vi "AppendToParentsList.vi"(10 "Dependendent TypeDefs wParents (in)":T1[](array[typedef]), 11 "Dependendent TypeDef wParents":T1) -> (2 "Dependendent TypeDefs wParents (out)":T1[](array[typedef]))   [LabVIEW 2013, in "DiscoverCommonTypeDefCallers.lvlib"]
uses:
  DiscoverCommonTypeDefCallers.lvlib
  DependendentTypeDefswParents.ctl
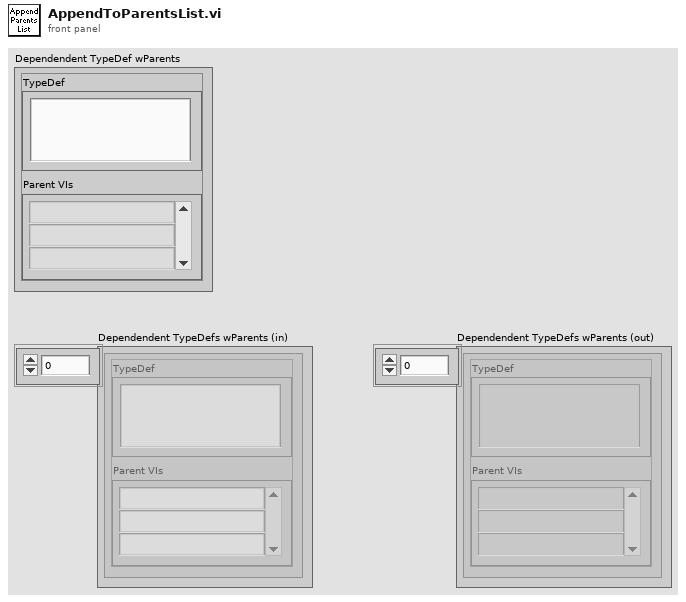
[diagram p1: front panel]
types:
  T1 = typedef "DiscoverCommonTypeDefCallers.lvlib/DependendentTypeDefswParents.ctl" = cluster{"TypeDef":string, "Parent VIs":string[]}
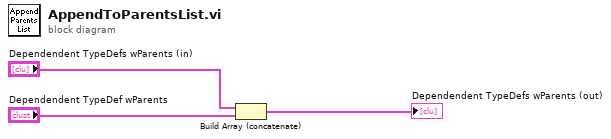
[diagram p0: block diagram]
diagram:
  n1 = Build Array (concatenate)("Dependendent TypeDefs wParents (in)", "Dependendent TypeDef wParents") -> (→"Dependendent TypeDefs wParents (out)":T1[])
